vi "ge_FindModProps.vi"(6 "Hdr Name":T2, 8 "error in (no error)":errorcluster, 9 "Device":string, 10 "MeasType":T1, 11 "All Ring Support":variant) -> (0 "error out":errorcluster, 3 "Values":u16[](array[numeric]))   [LabVIEW 2018]
uses:
  Common/Controls/HeaderNames.ctl
  Custom Ctrls/ge_MeasType.ctl
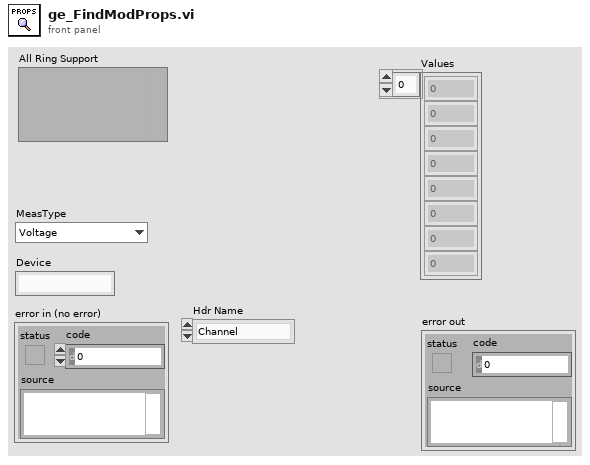
[diagram p1: front panel]
types:
  T1 = typedef "ge_MeasType.ctl" = enum16{"Voltage", "Frequency", "Tachometer", "Dynamic", "Thermocouple", "RTD", "Strain", "Current", "Resistance"}
  T2 = typedef "HeaderNames.ctl" = enum16{"Channel", "Device", "Spacer", "Description", "MB", "Range", "Terminal", "Coupling", "Thresh (V)", "Pulse/Rev", "Slope", "Min EU", "Min RPM", "mV/EU", "Iex", "Temp Units", "Type", "CJC Src", "CJC Val", "Ro", "Wire Cfg", "Strain Mode", "Vex", "Bridge Type", "GF", "Gauge Res", "Poisson", "Lead Res", "Init Strain", "GAF", "Scale", "Offset", "Unit (EU)", "dB?", "dB Ref", "Cal Mag", "Cal Units", "Max Temp", "Min Temp", "Max Strain", "Min Strain"}
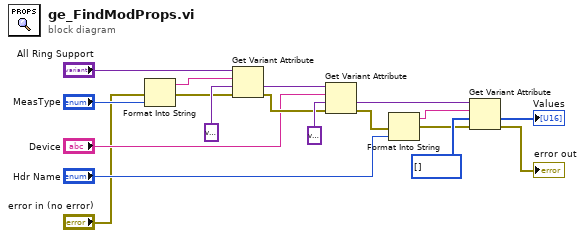
[diagram p0: block diagram]
diagram:
  n1 = Format Into String(error in="error in (no error)", "MeasType") -> (resulting string=w3:string, error out=w2:errorcluster)  [unwired: 2 in]
  n2 = Get Variant Attribute(Variant="All Ring Support", name=w3, default value (empty Variant)=variant ("All Ring Support"), error in=w2) -> (value=w1:variant, error out=w10:errorcluster)  [unwired: 2 out]
  n3 = Get Variant Attribute(Variant=w1, name="Device", default value (empty Variant)=variant ("All Ring Support"), error in=w10) -> (value=w8:variant, error out=w12:errorcluster)  [unwired: 2 out]
  n4 = Format Into String(error in=w12, "Hdr Name") -> (resulting string=w13:string, error out=w11:errorcluster)  [unwired: 2 in]
  n5 = Get Variant Attribute(Variant=w8, name=w13, default value (empty Variant)=u16[] [] ("Values"), error in=w11) -> (value=→"Values":u16[], error out=→"error out":errorcluster)  [unwired: 2 out]
